vi "reshape array (Ballard-1553).vi"(10 "size requested":i32=2, 11 "Array in":T1[](array[typedef])) -> (3 "Array out":T1[](array[typedef]))   [LabVIEW 2020]
uses:
  1553/_controls/ballard1553_cluster.ctl
  1553/_controls/aim1553_messages.ctl
  1553/_controls/1553_Parameters_key.ctl
  1553/_controls/1553_Parameters.ctl
  1553/_controls/1553_minorFrames.ctl
  1553/_controls/aim1553_cluster.ctl
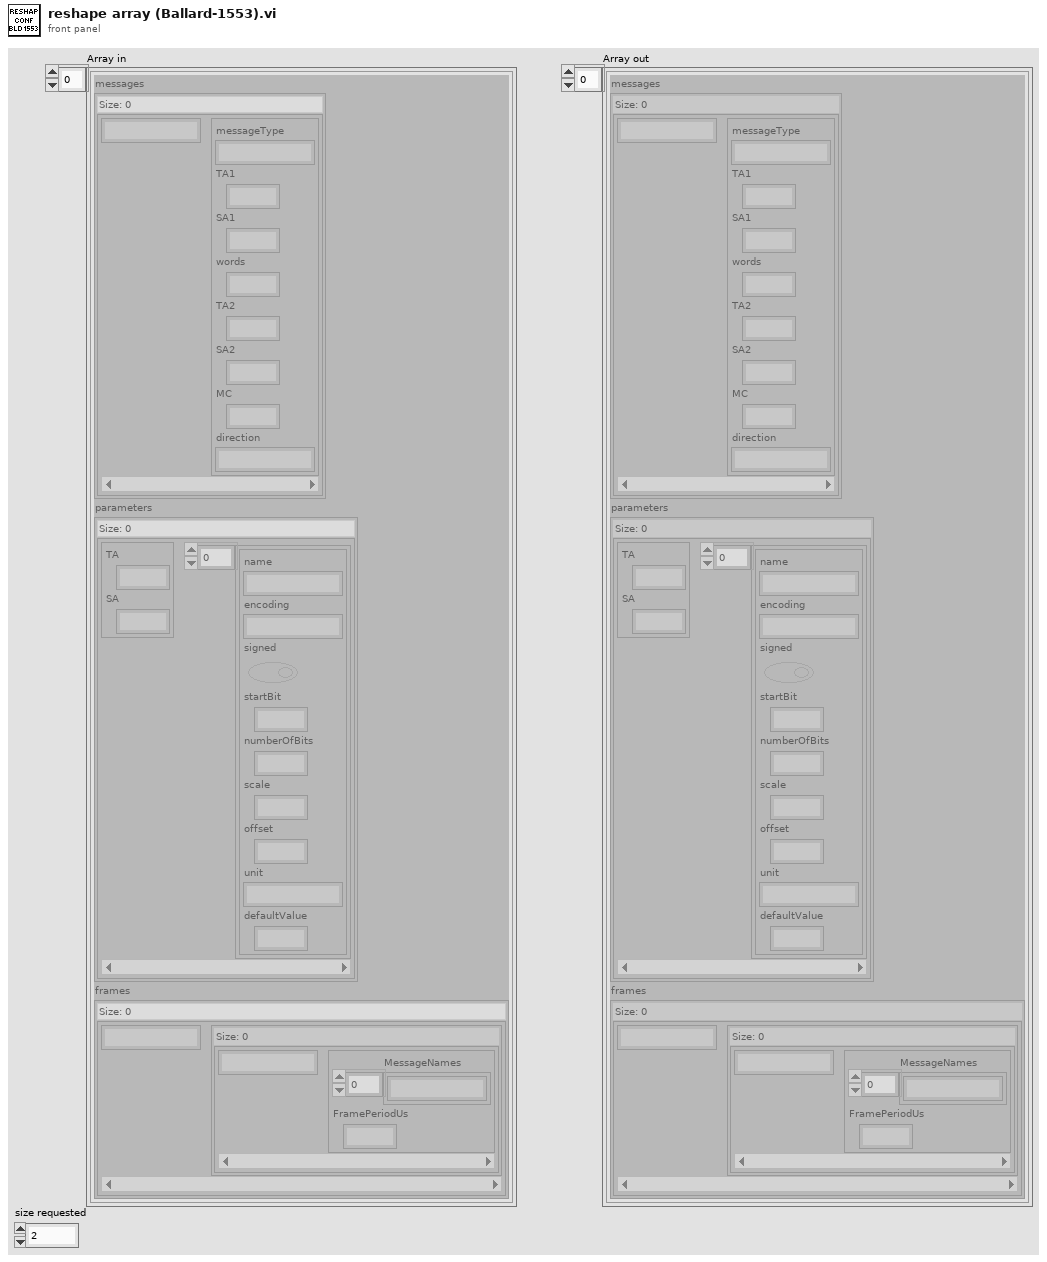
[diagram p1: front panel]
types:
  T1 = typedef "ballard1553_cluster.ctl" = cluster{"messages":map{string, T2}, "parameters":map{T3, T4[]}, "frames":map{string, map{string, T5}}}
  T2 = typedef "aim1553_messages.ctl" = cluster{"messageType":string, "TA1":i32, "SA1":i32, "words":i32, "TA2":i32, "SA2":i32, "MC":i32, "direction":string}
  T3 = typedef "1553_Parameters_key.ctl" = cluster{"TA":i32, "SA":i32}
  T4 = typedef "1553_Parameters.ctl" = cluster{"name":string, "encoding":string, "signed":bool, "startBit":i32, "numberOfBits":i32, "scale":dbl, "offset":dbl, "unit":string, "defaultValue":dbl}
  T5 = typedef "1553_minorFrames.ctl" = cluster{"MessageNames":string[], "FramePeriodUs":i32}
  T6 = typedef "aim1553_cluster.ctl" = cluster{"messages":map{string, T2}, "parameters":map{T3, T4[]}, "frames":map{string, map{string, T5}}}
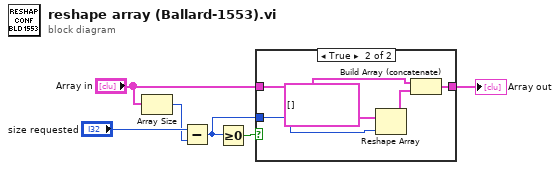
[diagram p0: block diagram]
diagram:
  n1 = Array Size(array="Array in") -> (size(s)=w5:i32)
  n2 = Subtract(x="size requested", y=w5) -> (x-y=w3:i32)
  n3 = Greater Or Equal To 0?(x=w3) -> (x >= 0?=w4:bool)
  n4 = case shown="True" w4 {
    tunnel: w3 -> [_ w11]
    tunnel: "Array in" -> [w7 w9]
    tunnel: [w7 w8] -> w1
    frame False {
    }
    frame True {
      n5 = Reshape Array(T6[] [] ("Array in"), w11) -> (w10:T6[])
      n6 = Build Array (concatenate)(w9, w10) -> (w8:T6[])
    }
  }
  "Array out" <- w1
